vi "计算误差.vi"(8 "反馈数值":sgl[][](array[numeric]), 11 "输入数值":sgl[][](array[numeric])) -> (1 "合格":bool[][](array[boolean]), 3 "误差":sgl[][](array[numeric]))   [LabVIEW 2010]
uses:
  全局量/全局_配置.vi
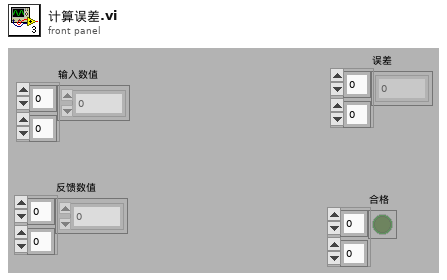
[diagram p1: front panel]
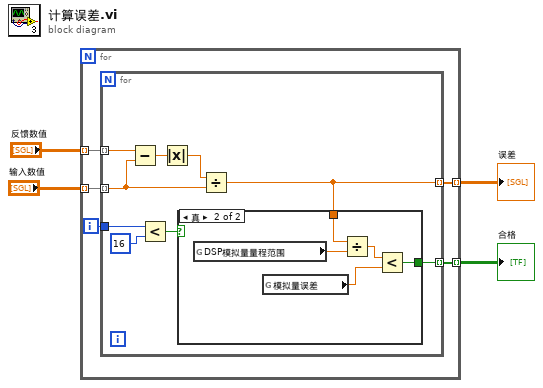
[diagram p0: block diagram]
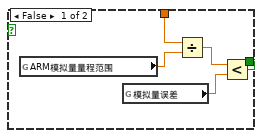
[diagram p2: hidden frame]
diagram:
  n1 = for {
    tunnel: "反馈数值" -> [w9] mode=indexing
    tunnel: "输入数值" -> [w8] mode=indexing
    tunnel: [w7] -> w2 mode=indexing
    tunnel: [w5] -> w1 mode=indexing
    i -> [w6]
    n2 = for {
      tunnel: w9 -> [w18] mode=indexing
      tunnel: w8 -> [w15] mode=indexing
      tunnel: [w11] -> w7 mode=indexing
      tunnel: w6 -> [w14]
      tunnel: [w10] -> w5 mode=indexing
      n3 = Subtract(x=w18, y=w15) -> (x-y=w17:sgl)
      n4 = Less?(x=w14, y=16) -> (x < y?=w12:bool)
      n5 = Absolute Value(x=w17) -> (abs(x)=w16:sgl)
      n6 = Divide(x=w16, y=w15) -> (x/y=w11:sgl)
      n7 = case shown="真" w12 {
        tunnel: w11 -> [w23 w28]
        tunnel: [w19 w24] -> w10
        frame False {
          n8 = global read "全局_配置.vi" "ARM模拟量量程范围"() -> (w22:sgl)
          n9 = global read "全局_配置.vi" "模拟量误差"() -> (w20:sgl)
          n10 = Divide(x=w23, y=w22) -> (x/y=w21:sgl)
          n11 = Less?(x=w21, y=w20) -> (x < y?=w19:bool)
        }
        frame True {
          n12 = global read "全局_配置.vi" "DSP模拟量量程范围"() -> (w27:sgl)
          n13 = global read "全局_配置.vi" "模拟量误差"() -> (w25:sgl)
          n14 = Divide(x=w28, y=w27) -> (x/y=w26:sgl)
          n15 = Less?(x=w26, y=w25) -> (x < y?=w24:bool)
        }
      }
    }
  }
  "误差" <- w2
  "合格" <- w1
